vi "Generate_Report_OLD_notes.vi"() -> ()   [LabVIEW 2020]
uses:
  <vilib>/Utility/NIReport.llb/Report Type.ctl
  <vilib>/Utility/NIReport.llb/NI_ReportGenerationCore.lvlib
  <vilib>/Utility/NIReport.llb/NI_report.lvclass
  <vilib>/Utility/NIReport.llb/Append Text Table to Report (wrap).vi
  <vilib>/Utility/NIReport.llb/Excel/NI_Excel.lvclass
panel:
  out "T button?":bool
  in  "Input Voltage":dbl
  out "error out":errorcluster
  in  "Min Voltage":dbl
  in  "Max Voltage":dbl
  in  "error in (no error)":errorcluster
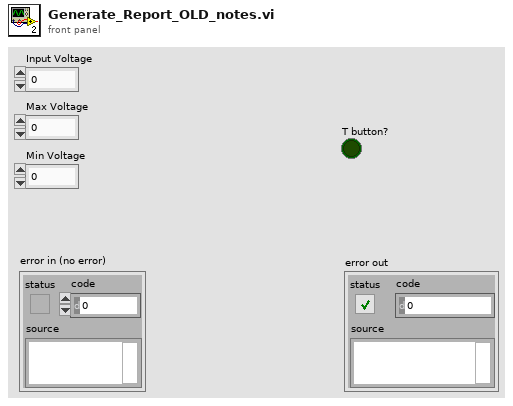
[diagram p1: front panel]
types:
  T1 = typedef "NI_ReportGenerationCore.lvlib/Report Type.ctl" = enum16{"HTML", "Word", "Excel"}
  T2 = cluster{"position (excel)":cluster{"row":i32, "column":i32}, "name (excel)":string, "bookmark (word)":string}
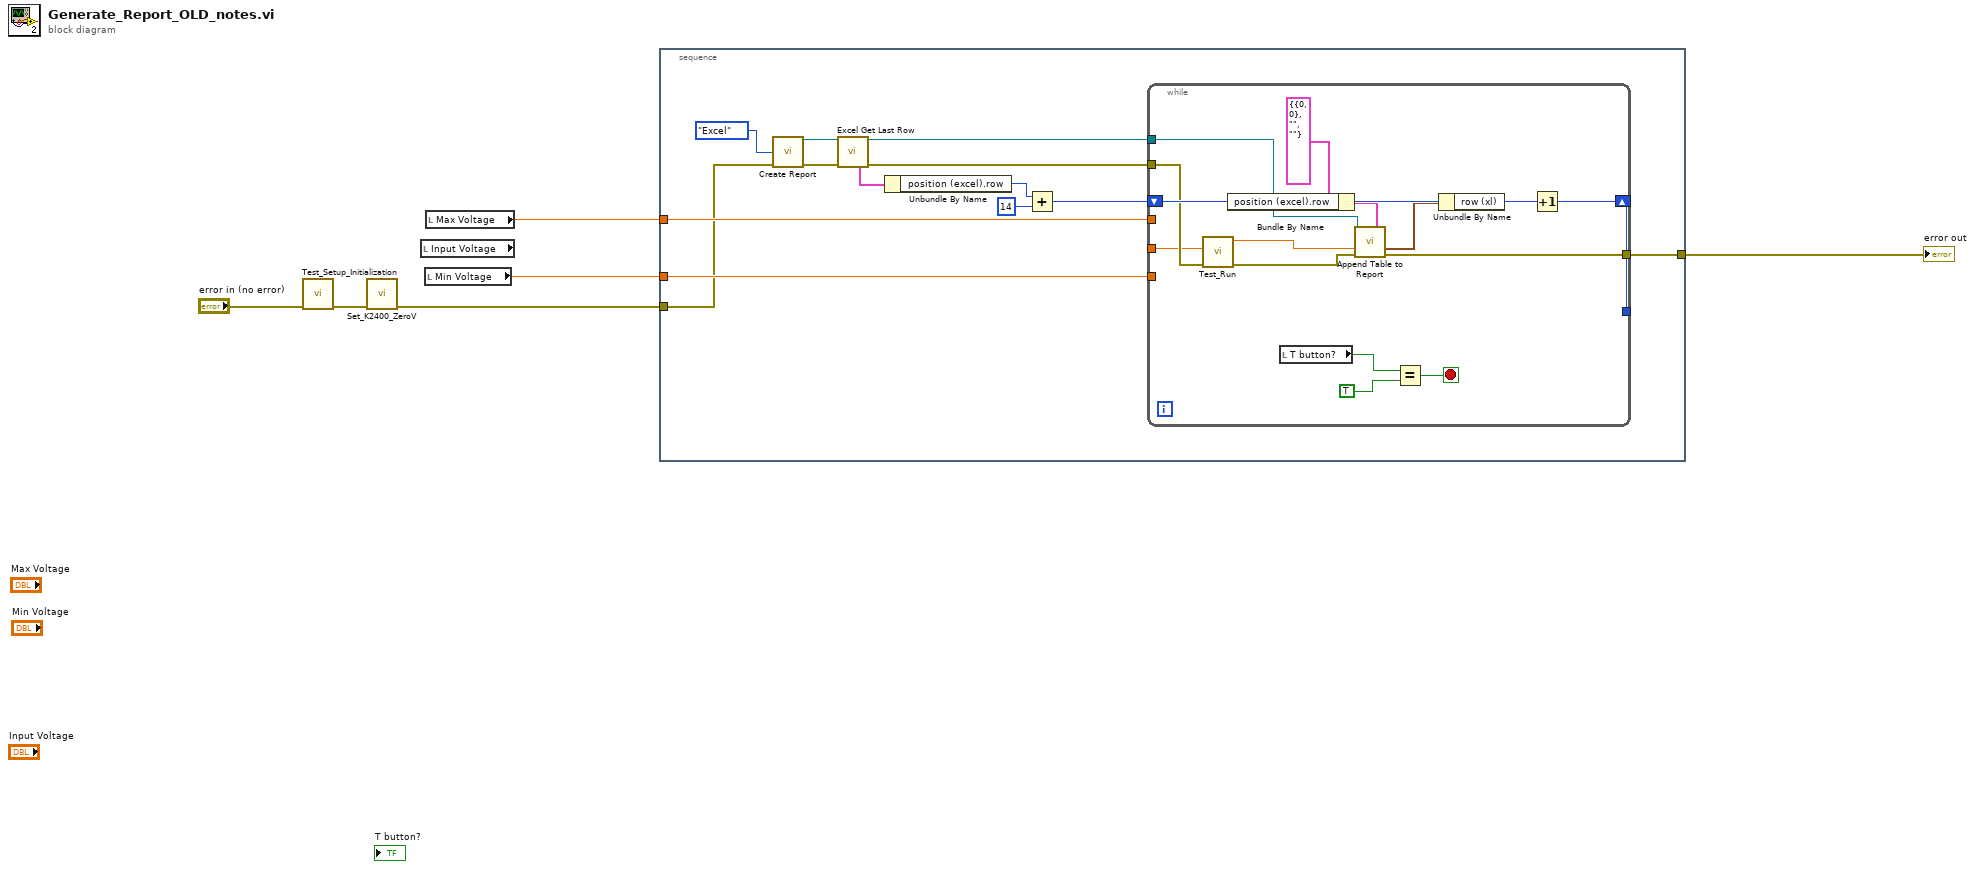
[diagram p0: block diagram]
diagram:
  n1 = call "Test_Setup_Initialization.vi"("HP 3457A Error In"="error in (no error)") -> ("HP 3457A Error Out"=w5:errorcluster)  [unwired: 10 in]
  n2 = call "Set_K2400_ZeroV.vi"("error in"=w5) -> ("error out"=w3:errorcluster)  [unwired: 10 in]
  n3 = local read "Input Voltage"() -> ()  [unwired: 1 out]
  n4 = local read "Min Voltage"() -> (w2:dbl)
  n5 = local read "Max Voltage"() -> (w1:dbl)
  n6 = stacked-sequence {
    tunnel: w2 -> [w19]
    tunnel: [w18] -> w6
    tunnel: w3 -> [w7]
    tunnel: w1 -> [w8]
    frame #0 {
      n7 = call <vilib>:"Create Report.vi"("report type"=Report_Type."Excel", "error in (no error)"=w7) -> ("report out"=w13:refnum<class "NI_report.lvclass">, "error out"=w11:errorcluster)  [unwired: 12 in]
      n8 = call <vilib>:"Excel Get Last Row.vi"("report in"=w13, "error in (no error)"=w11) -> ("report out"=w9:refnum<class "NI_report.lvclass">, "MS Office parameters out"=w15:T2, "error out"=w10:errorcluster)  [unwired: 11 in]
      n9 = Unbundle By Name(w15) -> ("position (excel).row"=w16:i32)
      n10 = Add(x=w16, y=14) -> (x+y=w12:i32)
      n11 = while {
        tunnel: w19 -> [_]
        shift-right: [w27] -> _
        shift-left: _ -> [w26]
        tunnel: [w24] -> w18
        tunnel: w12 -> [_]
        tunnel: w10 -> [w23]
        tunnel: w9 -> [w22]
        tunnel: w8 -> [_]
        tunnel: _ -> [w21]
        stop <- w33 stop-if-true
        n12 = call "Test_Run.vi"("error in"=w23, "Desired Voltage"=w21) -> ("error out"=w32:errorcluster, "Capacitance Data (in pF)"=w20:dbl)  [unwired: 6 in, 2 out]
        n13 = Bundle By Name(cluster=T2 {"position (excel)"={"row"=0, "column"=0}, "name (excel)"="", "bookmark (word)"=""} ("MS Office parameters"), "position (excel).row"=w26) -> (w30:T2)
        n14 = local read "T button?"() -> (w25:bool)
        n15 = call-poly <vilib>:"Append Table to Report.vi"("report in"=w22, "MS Office parameters"=w30, "text data"=w20, "error in (no error)"=w32) -> ("end (xl)"=w29:cluster{"row (xl) ":i32, "col (xl) ":i32}, "error out"=w24:errorcluster)  [unwired: 8 in, 2 out]
        n16 = Equal?(x=w25, y=TRUE) -> (x = y?=w33:bool)
        n17 = Unbundle By Name(w29) -> ("row (xl)"=w28:i32)
        n18 = Increment(x=w28) -> (x+1=w27:i32)
      }
    }
  }
  "error out" <- w6
